vi "Drive SS Safety 2016.vi"(10 "Drive Actuator Values In":T1) -> (2 "Drive Actuator Values Out":T1)   [LabVIEW 2015]
uses:
  Drive Actuator Values Out.ctl
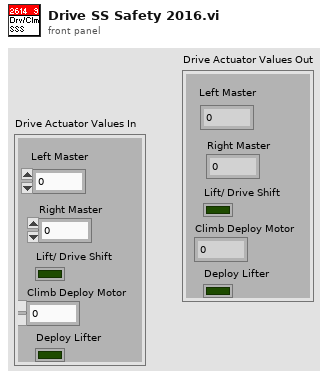
[diagram p1: front panel]
types:
  T1 = typedef "Drive Actuator Values Out.ctl" = cluster{"Left Master":dbl, "Right Master":dbl, "Lift/ Drive Shift":bool, "Climb Deploy Motor":dbl, "Deploy Lifter":bool}
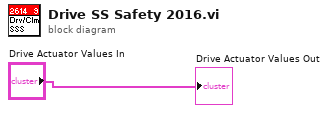
[diagram p0: block diagram]
diagram:
  "Drive Actuator Values Out" <- "Drive Actuator Values In"
